vi "Create.vi"(8 "ErrorIn":errorcluster, 11 "ReferenceIn":refnum<class "UserManager.lvclass">) -> (0 "ErrorOut":errorcluster, 3 "ReferenceOut":refnum<class "UserManager.lvclass">)   [LabVIEW 2021, in "UserMananger.lvlib" / "UserManager.lvclass"]
uses:
  UserManager.lvclass
  UserManager.lvclass/UserManager.ctl
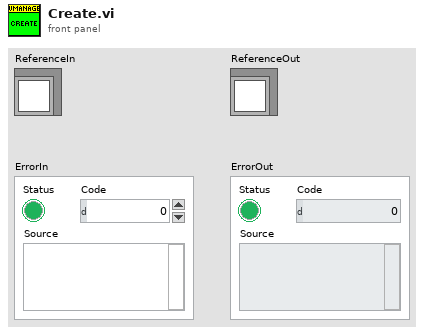
[diagram p1: front panel]
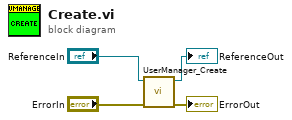
[diagram p0: block diagram]
diagram:
  n1 = call "UserManager_Create.vi"("ErrorIn"="ErrorIn", "ReferenceIn"="ReferenceIn") -> ("ErrorOut"=→"ErrorOut":errorcluster, "ReferenceOut"=→"ReferenceOut":refnum<class "UserManager.lvclass">)  [unwired: 8 in]
